vi "array_select.vi"(10 "Selection":i32[](array[numeric]), 11 "Array In":string[](array[string])) -> (3 "Array Out":string[](array[string]))   [LabVIEW 2018]
doc: "Reduces the Input Array to the elements specified in N."
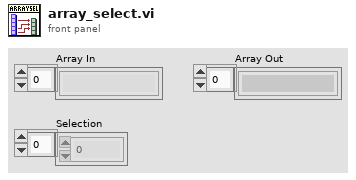
[diagram p1: front panel]
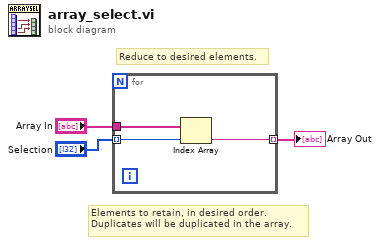
[diagram p0: block diagram]
diagram:
  # "Elements to retain, in desired order.\nDuplicates will be duplicated in the array."
  # "Reduce to desired elements."
  n1 = for {
    tunnel: "Selection" -> [w5] mode=indexing
    tunnel: "Array In" -> [w6]
    tunnel: [w4] -> w3 mode=indexing
    n2 = Index Array(array=w6, index=w5) -> (element=w4:string)
  }
  "Array Out" <- w3
